vi "List Measurements.vi"(8 "error in (no error)":errorcluster, 10 "Channel (1)":i32=1, 11 "VISA resource name":refnum<visa-resource-name>) -> (0 "error out":errorcluster, 1 "Measurement Parameters":string[](array[string]), 2 "Measurement Names":string[](array[string]), 3 "VISA resource name out":refnum<visa-resource-name>)   [LabVIEW 2018, in "Keysight PNA Series.lvlib"]
doc: "Returns the names and parameters of existing measurements for the specified channel."
uses:
  Keysight PNA Series.lvlib
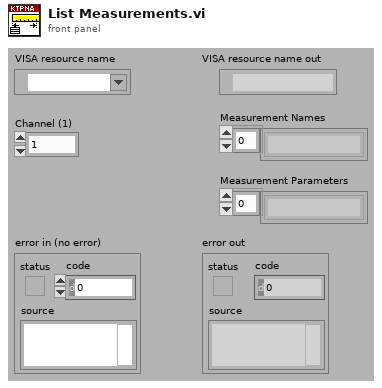
[diagram p1: front panel]
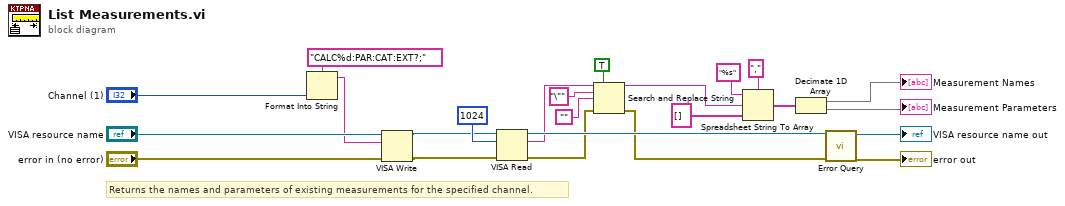
[diagram p0: block diagram]
diagram:
  # "Returns the names and parameters of existing measurements for the specified channel."
  n1 = Format Into String(format string="CALC%d:PAR:CAT:EXT?;", "Channel (1)") -> (resulting string=w8:string)  [unwired: 2 in, 1 out]
  n2 = VISA Write(VISA resource name="VISA resource name", write buffer=w8, error in (no error)="error in (no error)") -> (VISA resource name out=w11:refnum<visa-resource-name>, error out=w10:errorcluster)  [unwired: 1 out]
  n3 = VISA Read(VISA resource name=w11, byte count=u32 1024, error in (no error)=w10) -> (VISA resource name out=w9:refnum<visa-resource-name>, read buffer=w7:string, error out=w2:errorcluster)  [unwired: 1 out]
  n4 = Search and Replace String(replace all?=TRUE ("replace all? (F)"), input string=w7, search string="\"", replace string="", error in=w2) -> (result string=w4:string, error out=w1:errorcluster)  [unwired: 3 in, 2 out]
  n5 = Spreadsheet String To Array(delimiter (Tab)=",", format string="%s", spreadsheet string=w4, array type (2D Dbl)=string[] []) -> (array=w14:string[])
  n6 = Decimate 1D Array(w14) -> (→"Measurement Names":string[], →"Measurement Parameters":string[])
  n7 = call "Error Query.vi"("error in (no error)"=w1, "VISA resource name"=w9) -> ("error out"=→"error out":errorcluster, "VISA resource name out"=→"VISA resource name out":refnum<visa-resource-name>)  [unwired: 6 in, 2 out]
